vi "Konvolucio MUDS150628 B232EATC Read DTC TesterPresent.vi"() -> ()   [LabVIEW 2011]
uses:
  <instrlib>/Konvolucio MUDS150628/Types/DtcItemType.ctl
  <instrlib>/Konvolucio MUDS150628/Konvolucio MUDS150628.lvlib
panel:
  out "DtcItems":T1[](array[typedef])
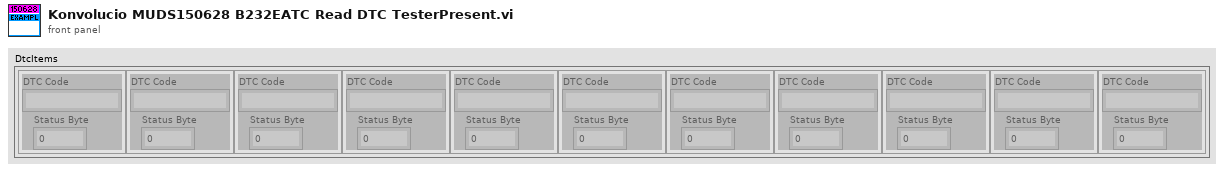
[diagram p1: front panel]
types:
  T1 = typedef "Konvolucio MUDS150628.lvlib/DtcItemType.ctl" = cluster{"DTC Code":string, "Status Byte":i32}
  T2 = typedef "Konvolucio MUDS150628.lvlib/UdsHandleType.ctl" = cluster{"LogPath":path, "LogEnabled":bool, "isOpen":bool, "LogContent":string, "Adapter":string, "MCanHandle":T3, "TransmittId":u32, "ReceiveId":u32}
  T3 = typedef "Konvolucio MCAN120803.lvlib/MCanHandleType.ctl" = cluster{"MCanAdapter":refnum<k24>}
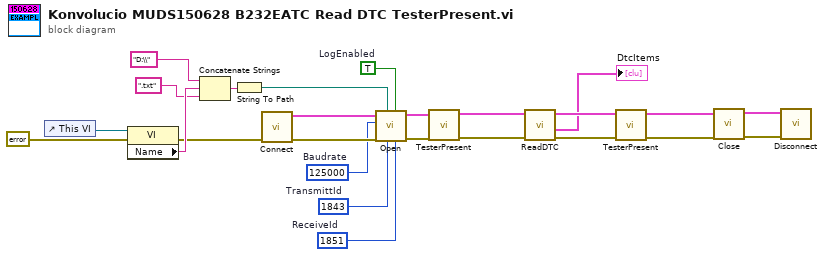
[diagram p0: block diagram]
diagram:
  w8 = TRUE  # LogEnabled
  w7 = u32 125000  # Baudrate
  w4 = u32 1851  # ReceiveId
  w5 = u32 1843  # TransmittId
  n1 = control-ref of="This VI"() -> (w16:refnum<vi>)
  n2 = property class="VI"(reference=w16, error in=errorcluster {"status"=FALSE, "code"=0, "source"=""} ("error in (no error)")) -> (error out=w11:errorcluster, "Name"=w14:string)  [unwired: 1 out]
  n3 = Concatenate Strings("D:\\" ("VI Name"), w14, ".txt" ("string")) -> (w12:string)
  n4 = String To Path(string=w12) -> (path=w6:path)
  n5 = call <instrlib>:"Connect.vi"("error in"=w11) -> ("error out"=w9:errorcluster, "UdsHandleOut"=w10:T2)  [unwired: 9 in]
  n6 = call <instrlib>:"Open.vi"("ReceiveId"=w4, "LogEnabled"=w8, "TransmittId"=w5, "LogPath"=w6, "error in"=w9, "BaudRate"=w7, "UdsHandleIn"=w10) -> ("error out"=w2:errorcluster, "UdsHandleOut"=w1:T2)  [unwired: 3 in]
  n7 = call <instrlib>:"TesterPresent.vi"("error in"=w2, "UdsHandleIn"=w1) -> ("error out"=w25:errorcluster, "UdsHandleOut"=w24:T2)  [unwired: 8 in]
  n8 = call <instrlib>:"ReadDTC.vi"("error in"=w25, "UdsHandleIn"=w24) -> ("error out"=w23:errorcluster, "DtcItems"=→"DtcItems":T1[], "UdsHandleOut"=w22:T2)  [unwired: 6 in, 1 out]
  n9 = call <instrlib>:"TesterPresent.vi"("error in"=w23, "UdsHandleIn"=w22) -> ("error out"=w21:errorcluster, "UdsHandleOut"=w20:T2)  [unwired: 8 in]
  n10 = call <instrlib>:"Close.vi"("error in"=w21, "UdsHandleIn"=w20) -> ("error out"=w18:errorcluster, "UdsHandleOut"=w17:T2)  [unwired: 8 in]
  n11 = call <instrlib>:"Disconnect.vi"("error in"=w18, "UdsHandleIn"=w17) -> ()  [unwired: 9 in, 1 out]
